vi "Check Read Complete (SubVI).vi"(11 "JSON String":string) -> (3 "Complete?":bool)   [LabVIEW 2015]
uses:
  Library/Token.ctl
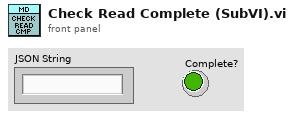
[diagram p1: front panel]
types:
  T1 = typedef "Token.ctl" = enum16{"End", "Boolean", "Named Cluster", "Unnamed Cluster", "Array", "String", "Decimal", "FloatingPoint", "End Array", "End Cluster"}
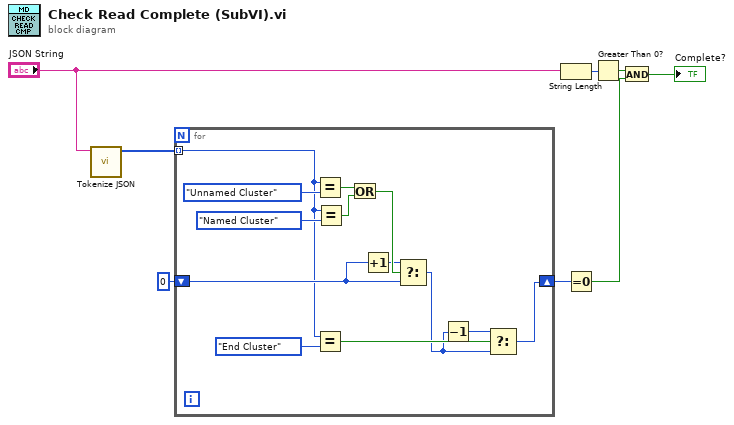
[diagram p0: block diagram]
diagram:
  n1 = call "Tokenize JSON.vi"("JSON String"="JSON String") -> ("Token Array"=w5:T1[])  [unwired: 9 in, 1 out]
  n2 = for {
    tunnel: w5 -> [w13] mode=indexing
    shift-right: [w9] -> w7
    shift-left: 0 -> [w15]
    n3 = Equal?(x=w13, y=Token."Unnamed Cluster") -> (x = y?=w19:bool)
    n4 = Equal?(x=w13, y=Token."End Cluster") -> (x = y?=w12:bool)
    n5 = Equal?(x=w13, y=Token."Named Cluster") -> (x = y?=w18:bool)
    n6 = Or(x=w19, y=w18) -> (x .or. y?=w17:bool)
    n7 = Increment(x=w15) -> (x+1=w16:i32)
    n8 = Select(t=w16, s=w17, f=w15) -> (s? t:f=w11:i32)
    n9 = Decrement(x=w11) -> (x-1=w10:i32)
    n10 = Select(t=w10, s=w12, f=w11) -> (s? t:f=w9:i32)
  }
  n11 = String Length(string="JSON String") -> (length=w4:i32)
  n12 = Equal To 0?(x=w7) -> (x = 0?=w8:bool)
  n13 = Greater Than 0?(x=w4) -> (x > 0?=w1:bool)
  n14 = And(x=w1, y=w8) -> (x .and. y?=→"Complete?":bool)
